vi "DrawCircle.vi"(7 "Color":T2, 8 "Radius":u32, 9 "Center coord":u32[](array[numeric]), 10 "New Image":T1, 11 "Refnum in":T1) -> (3 "Refnum out":T1)   [LabVIEW 2024]
uses:
  <vilib>/vision/Image Controls.llb/IMAQ Image.ctl
  <vilib>/vision/NI_Vision_Development_Module.lvlib
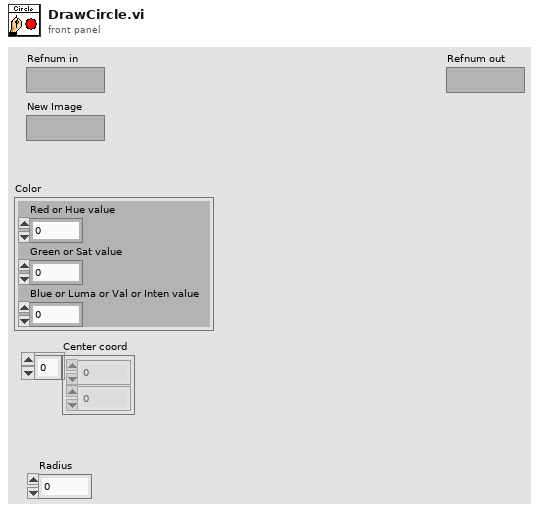
[diagram p1: front panel]
types:
  T1 = typedef "IMAQ Image.ctl" = refnum<image>
  T2 = cluster{"Red or Hue value":u8, "Green or Sat value":u8, "Blue or Luma or Val or Inten value":u8}
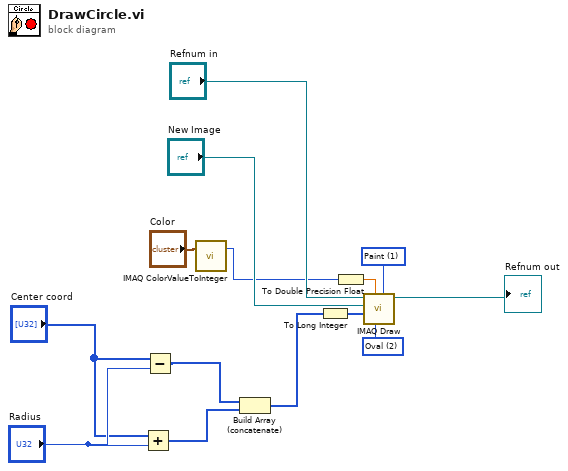
[diagram p0: block diagram]
diagram:
  w11 = u16 1 items=["Frame", "Paint", "Invert Frame", "Invert Paint"] ("Draw Mode")
  w10 = u16 2 items=["Line", "Rectangle", "Oval"] ("Shape to draw")
  n1 = Add(x="Center coord", y="Radius") -> (x+y=w5:u32[])
  n2 = Subtract(x="Center coord", y="Radius") -> (x-y=w6:u32[])
  n3 = call "IMAQ ColorValueToInteger"("Color Value"="Color") -> ("U32 value"=w3:u32)  [unwired: 4 in, 3 out]
  n4 = Build Array (concatenate)(w6, w5) -> (w4:u32[])
  n5 = To Long Integer(number=w4) -> (32bit integer=w2:i32[])
  n6 = To Double Precision Float(number=w3) -> (double precision float=w1:dbl)
  n7 = call "IMAQ Draw"("Draw Mode"=w11, "Shape to draw"=w10, "Pixel Color"=w1, "Coordinates"=w2, "Image Dst"="New Image", "Image Src"="Refnum in") -> ("Image Dst Out"=→"Refnum out":T1)  [unwired: 4 in, 1 out]
